vi "Waveform List cleanup.vi"() -> ()   [LabVIEW 2017, in "Waveform-Processing-Custom-Device System Explorer.lvlib"]
uses:
  Waveform-Processing-Custom-Device System Explorer.lvlib
  <userlib>/_OpenG.lib/array/array.llb/Remove Duplicates from 1D Array (String)__ogtk.vi
panel:
  out "Available Wavefroms Out":string[](array[string])
  in  "Removed Wavefroms":string[](array[string])
  in  "Available Wavefroms":string[](array[string])
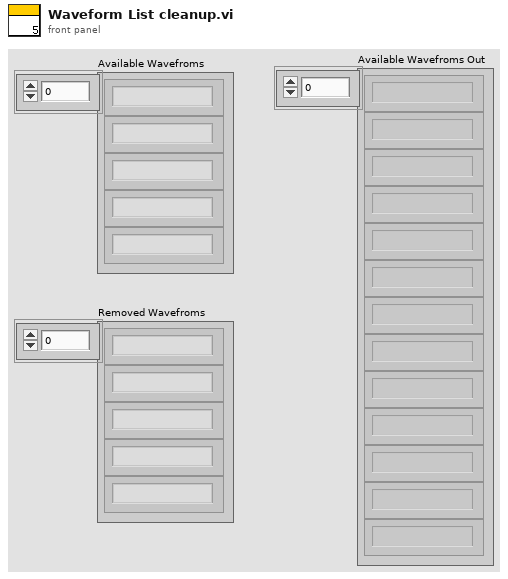
[diagram p1: front panel]
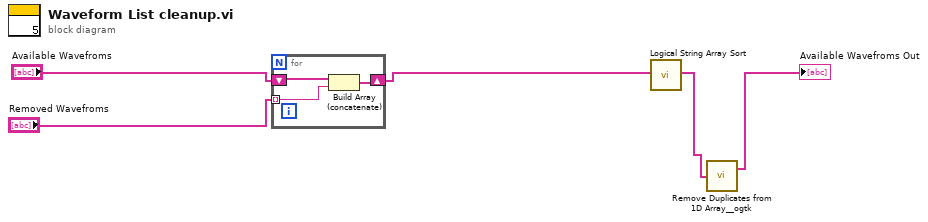
[diagram p0: block diagram]
diagram:
  n1 = for {
    tunnel: "Removed Wavefroms" -> [w7] mode=indexing
    shift-right: [w6] -> w1
    shift-left: "Available Wavefroms" -> [w8]
    n2 = Build Array (concatenate)(w8, w7) -> (w6:string[])
  }
  n3 = call "Logical String Array Sort.vi"("Unsorted List"=w1) -> ("Sorted List"=w5:string[])  [unwired: 18 in]
  n4 = call-poly <userlib>:"Remove Duplicates from 1D Array__ogtk.vi"("Input Array"=w5) -> ("Output Array"=→"Available Wavefroms Out":string[])  [unwired: 1 out]
